vi "Pattern Matching_Test.vi"(8 "error in (no error)":errorcluster, 9 "Template file path":path=path "D:/Focusing Station/Sub VIs/RH_Center_template.PNG", 10 "Image in":T1, 11 "File Path":path=path "C:/images/img1.jpeg") -> (0 "Image out":T1(plugin-control), 1 "y":sgl=579.59296, 2 "x":sgl=1185.8351, 3 "Pattern Presence":bool=TRUE, 4 "error out":errorcluster)   [LabVIEW 2019]
uses:
  <vilib>/vision/Pattern Matching.llb/IMAQ Pattern Match Advanced Options.ctl
  <vilib>/vision/Image Controls.llb/IMAQ Image.ctl
  <vilib>/vision/NI_Vision_Development_Module.lvlib
panel:
  out "Template":T1(plugin-control)
  out "Number of Matches Found":i32=1
  in  "Advanced Options":cluster{"Item":T2, "Value":dbl}[](array[cluster])=[{"Item"=1, "Value"=1.0}, {"Item"=103, "Value"=1.0}] {"Item" items=["LD Sampling - Minimum Constrast"=0, "LD Sampling - Enable Subpixel Accuracy"=1, "LD Sampling - Search Strategy"=2, "LD Sampling - Subpixel Iterations"=3, "LD Sampling - Subpixel Tolerance"=4, "LD Sampling - Initial Match List Length"=5, "LD Sampling - Match List Reduction Factor"=6, "LD Sampling - Initial Step Size"=7, "LD Sampling - Intermediate Angular Accuracy"=8, "-"=9, "Pyramid - Max Pyramid Level"=100, "Pyramid - Minimum Contrast"=102, "Pyramid - Enable Subpixel Accuracy"=103, "Pyramid - Subpixel Iterations"=104, "Pyramid - Subpixel Tolerance"=105, "Pyramid - Initial Match List Length"=106, "Pyramid - Match List Reduction Factor"=107, "Pyramid - Intermediate Angular Accuracy"=108, "Pyramid - Process Border Matches"=109, "Pyramid - Min Match Separation Distance"=111, "Pyramid - Min Match Separation Angle"=112, "Pyramid - Max Match Overlap"=113, "Pyramid - Max Cache in MB"=114, "Pyramid - Clear Cache"=115, "Pyramid - Enable Accurate Score Computation"=116, "Pyramid - Interpolation Method For Score Computation"=117, "Pyramid - Enable Target To Template Score"=118, "-"=119, "Enable Defect Map"=200]}
  in  "Match Parameters":T3={"Number of Matches Requested"=1, "Minimum Match Score"=750.0, "Angle Ranges"=[]} {"Angle Ranges"."End Angle" min=-360 max=360; "Angle Ranges"."Start Angle" min=-360 max=360; "Minimum Match Score" min=0 max=1000; "Number of Matches Requested" min=1 max=9999}
  out "Matches":T4(array[cluster])=[{"Position"={"x"=1185.8351, "y"=579.59296}, "Angle"=0.0, "Scale"=1.0, "Score"=892.4644, "Bounding Box"=[{"x"=1148.8351, "y"=542.59296}, {"x"=1222.8351, "y"=542.59296}, {"x"=1222.8351, "y"=616.59296}, {"x"=1148.8351, "y"=616.59296}, {"x"=1148.8351, "y"=542.59296}]}] {"Bounding Box"."y" format="%.2g"; "Bounding Box"."x" format="%.2g"; "Score" format="%.2f"; "Scale" format="%.2g"; "Angle" format="%.2g"; "Position"."y" format="%.2g"; "Position"."x" format="%.2g"}
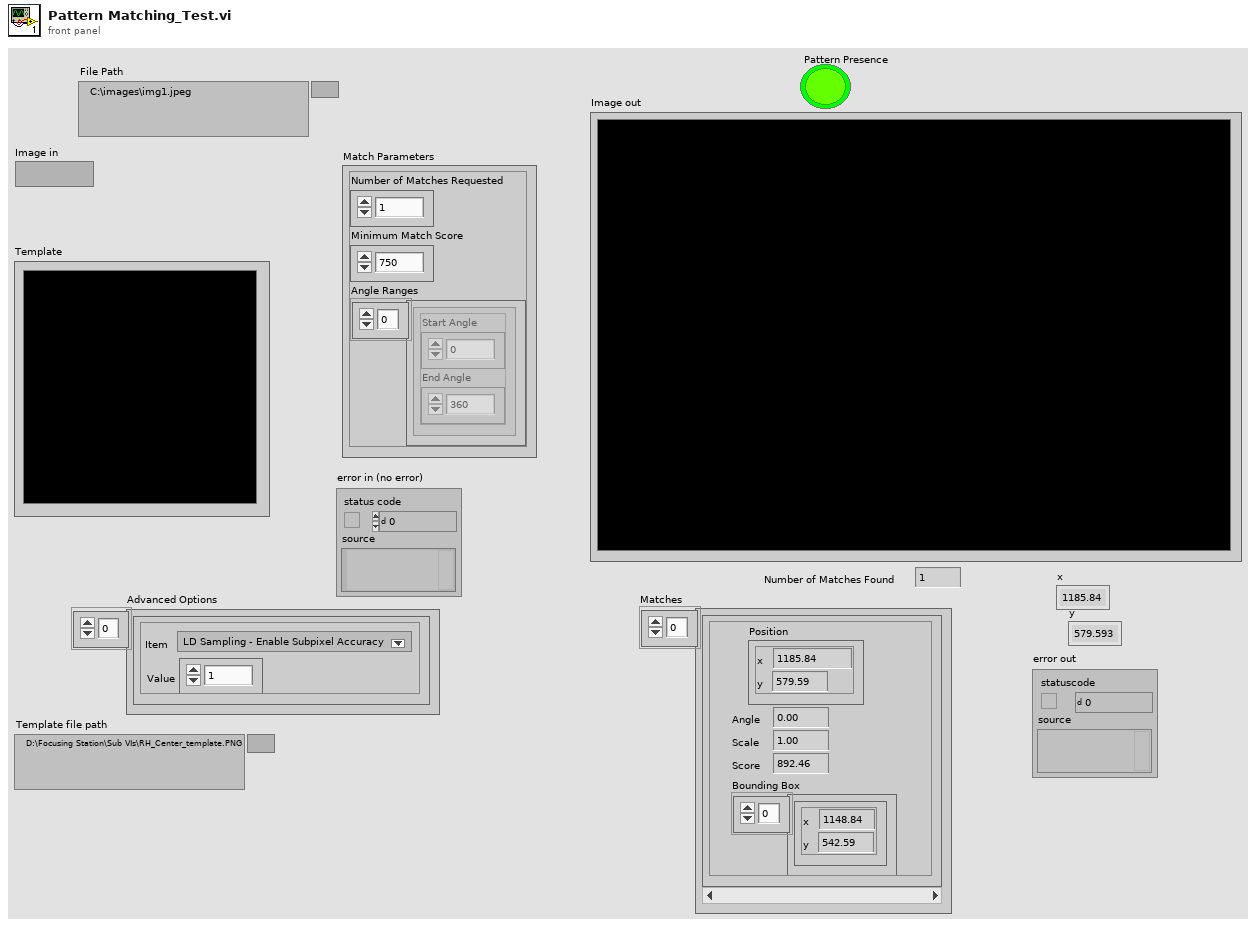
[diagram p1: front panel]
types:
  T1 = typedef "IMAQ Image.ctl" = refnum<image>
  T2 = typedef "IMAQ Pattern Match Advanced Options.ctl" = u16
  T3 = cluster{"Number of Matches Requested":i32, "Minimum Match Score":sgl, "Angle Ranges":cluster{"Start Angle":sgl, "End Angle":sgl}[]}
  T4 = cluster{"Position":cluster{"x":sgl, "y":sgl}, "Angle":sgl, "Scale":sgl, "Score":sgl, "Bounding Box":cluster{"x":sgl, "y":sgl}[]}[]
  T5 = typedef "Image Type" = u32
  T6 = cluster{"Position":cluster{"x":sgl, "y":sgl}, "Angle":sgl, "Scale":sgl, "Score":sgl, "Bounding Box":cluster{"x":sgl, "y":sgl}[]}
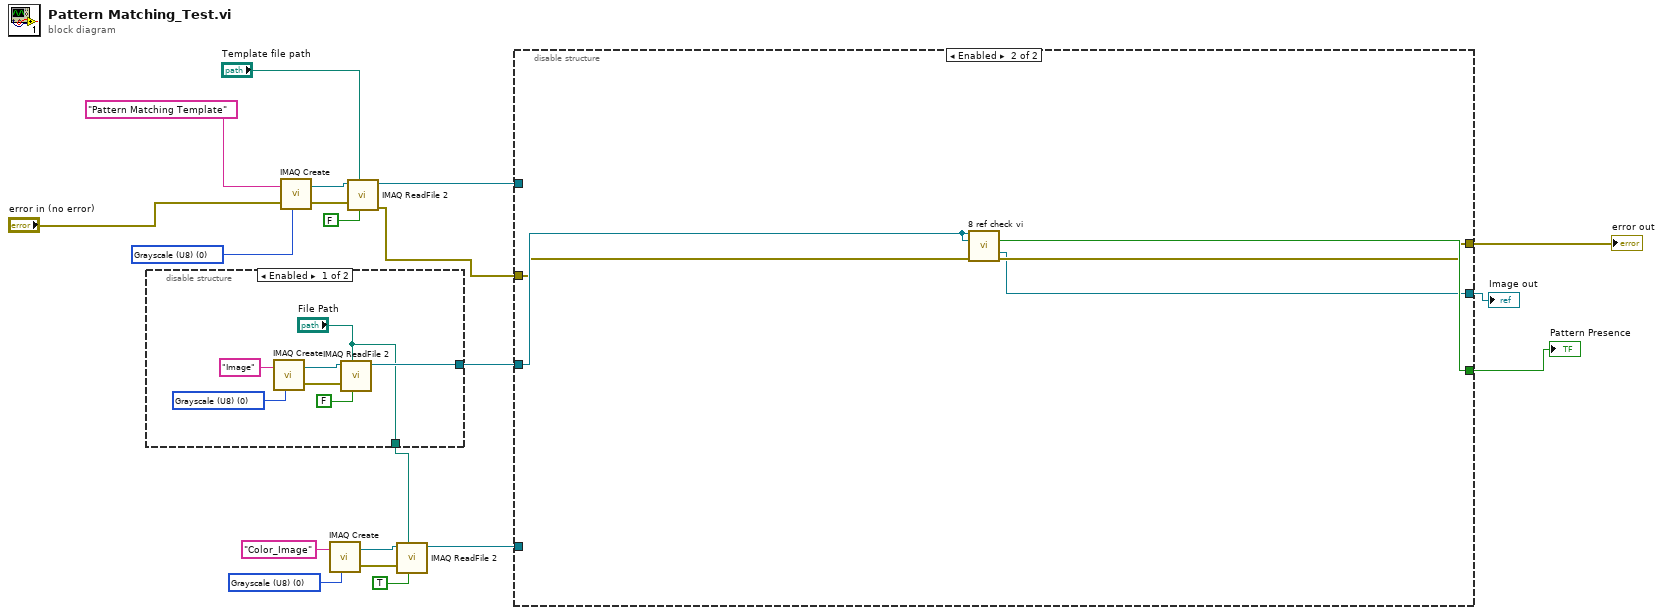
[diagram p0: block diagram]
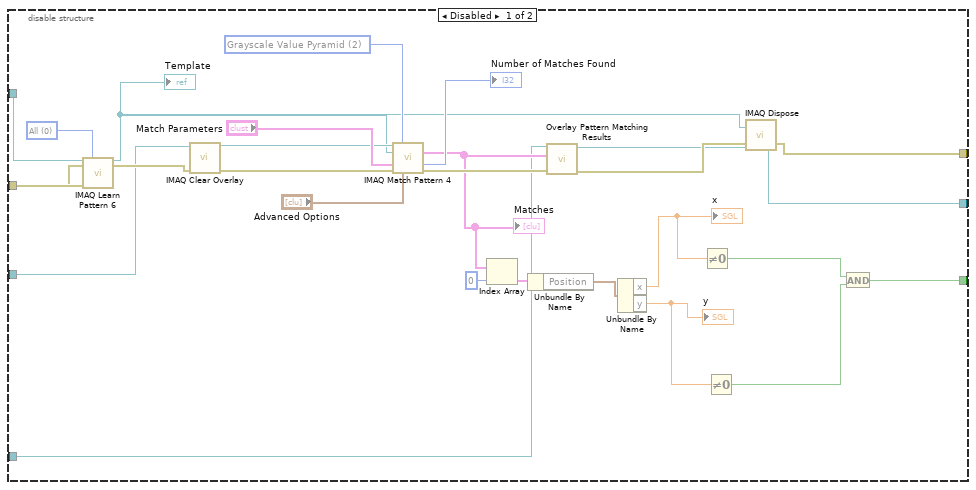
[diagram p2: hidden frame]
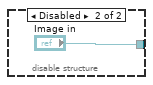
[diagram p3: hidden frame]
diagram:
  w6 = T5 0 items=["Grayscale (U8)", "Grayscale (I16)", "Grayscale (SGL)", "Complex (CSG)", "RGB (U32)", "HSL (U32)", "RGB (U64)", "Grayscale (U16)"] ("Image Type")
  w19 = T5 0 items=["Grayscale (U8)", "Grayscale (I16)", "Grayscale (SGL)", "Complex (CSG)", "RGB (U32)", "HSL (U32)", "RGB (U64)", "Grayscale (U16)"] ("Image Type")
  n1 = disable-structure shown="Enabled" {
    disable-tunnel: [w22 "Image in"] -> w13
    disable-tunnel: ["File Path" _] -> w4
    frame Enabled {
      w26 = T5 0 items=["Grayscale (U8)", "Grayscale (I16)", "Grayscale (SGL)", "Complex (CSG)", "RGB (U32)", "HSL (U32)", "RGB (U64)", "Grayscale (U16)"] ("Image Type")
      n2 = call "IMAQ Create"("Image Name"="Image", "Image Type"=w26) -> ("New Image"=w24:T1, "error out"=w23:errorcluster)  [unwired: 3 in]
      n3 = call "IMAQ ReadFile 2"("Use File Path Image Type"=FALSE, "File Path"="File Path", "error in (no error)"=w23, "Image"=w24) -> ("Image Out"=w22:T1)  [unwired: 3 in, 4 out]
    }
    frame Disabled {
    }
  }
  n4 = call "IMAQ Create"("Image Name"="Pattern Matching Template", "Image Type"=w19, "error in (no error)"="error in (no error)") -> ("New Image"=w17:T1, "error out"=w15:errorcluster)  [unwired: 2 in]
  n5 = call "IMAQ Create"("Image Name"="Color_Image", "Image Type"=w6) -> ("New Image"=w8:T1, "error out"=w9:errorcluster)  [unwired: 3 in]
  n6 = call "IMAQ ReadFile 2"("Use File Path Image Type"=FALSE, "File Path"="Template file path", "error in (no error)"=w15, "Image"=w17) -> ("error out"=w14:errorcluster, "Image Out"=w16:T1)  [unwired: 3 in, 3 out]
  n7 = call "IMAQ ReadFile 2"("Use File Path Image Type"=TRUE, "File Path"=w4, "error in (no error)"=w9, "Image"=w8) -> ("Image Out"=w3:T1)  [unwired: 3 in, 4 out]
  n8 = disable-structure shown="Enabled" {
    disable-tunnel: w16 -> [w53 _]
    disable-tunnel: w14 -> [w52 w57]
    disable-tunnel: w13 -> [w37 w59]
    disable-tunnel: [w32 w58] -> w12
    disable-tunnel: w3 -> [w31 _]
    disable-tunnel: [w30 w56] -> w2
    disable-tunnel: [w29 w55] -> w1
    frame Disabled {
      w51 = 2 items=["All", "Low Discrepancy Sampling", "Grayscale Value Pyramid", "Gradients Pyramid"] ("Algorithm")
      w54 = 0 items=["All", "Low Discrepancy Sampling", "Grayscale Value Pyramid", "Gradients Pyramid"] ("Algorithm")
      n9 = call "IMAQ Learn Pattern 6"("Image"=w53, "Algorithm"=w54, "error in (no error)"=w52) -> ("Template Image Out"=w42:T1, "error out"=w46:errorcluster)  [unwired: 10 in, 1 out]
      "Template" <- w42
      n10 = call "IMAQ Clear Overlay"("error in (no error)"=w46, "Image"=w37) -> ("error out"=w45:errorcluster, "Image Out"=w49:T1)  [unwired: 8 in]
      n11 = call "IMAQ Match Pattern 4"("Image"=w49, "Algorithm"=w51, "Template Image"=w42, "Parameters"="Match Parameters", "error in (no error)"=w45, "Advanced Options"="Advanced Options") -> ("Matches (pixel)"=w41:T4, "Number of Matches"=→"Number of Matches Found":i32, "error out"=w44:errorcluster)  [unwired: 5 in, 2 out]
      "Matches" <- w41
      n12 = Index Array(array=w41, index=0) -> (element=w39:T6)
      n13 = Unbundle By Name(w39) -> ("Position"=w38:cluster{"x":sgl, "y":sgl})
      n14 = call "Overlay Pattern Matching Results.vi"("error in"=w44, "Matches"=w41, "Image"=w31) -> ("error out"=w43:errorcluster, "Image Out"=w29:T1)  [unwired: 7 in]
      n15 = Unbundle By Name(w38) -> ("x"=w35:sgl, "y"=w36:sgl)
      "x" <- w35
      "y" <- w36
      n16 = Not Equal To 0?(x=w35) -> (x != 0?=w34:bool)
      n17 = Not Equal To 0?(x=w36) -> (x != 0?=w33:bool)
      n18 = call "IMAQ Dispose"("Image"=w42, "error in (no error)"=w43) -> ("error out"=w30:errorcluster)  [unwired: 4 in]
      n19 = And(x=w34, y=w33) -> (x .and. y?=w32:bool)
    }
    frame Enabled {
      n20 = call "8 ref check vi.vi"("Image In"=w59, "Image Dst"=w59, "error in"=w57) -> ("x = y?"=w58:bool, "Image Out 2"=w55:T1, "error out"=w56:errorcluster)  [unwired: 9 in, 1 out]
    }
  }
  "Pattern Presence" <- w12
  "error out" <- w2
  "Image out" <- w1
